vi "read_data.vi"(8 "error in (no error)":errorcluster, 11 "GammaRegressor in":refnum<class "GammaRegressor.lvclass">) -> (0 "error out":errorcluster, 2 "data":T1, 3 "GammaRegressor out":refnum<class "GammaRegressor.lvclass">)   [LabVIEW 2020, in "GammaRegressor.lvclass"]
uses:
  GammaRegressor.lvclass
  Controls/gamma_regressor_data.ctl
  GammaRegressor.lvclass/GammaRegressor.ctl
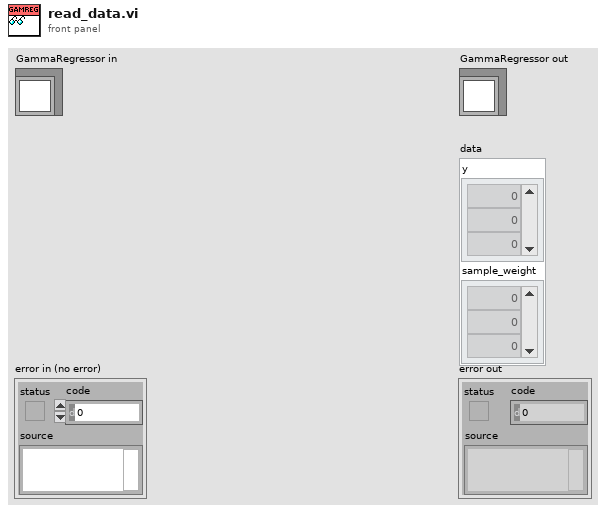
[diagram p1: front panel]
types:
  T1 = typedef "gamma_regressor_data.ctl" = cluster{"y":dbl[], "sample_weight":dbl[]}
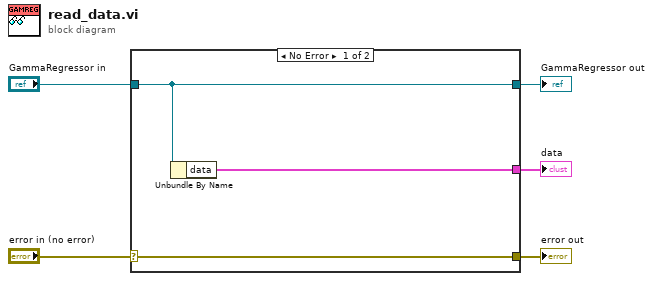
[diagram p0: block diagram]
diagram:
  n1 = case shown="No Error" "error in (no error)" {
    selector: "error in (no error)" -> [w8 w9]
    tunnel: [w8 w9] -> w4
    tunnel: [w7 w10] -> w2
    tunnel: "GammaRegressor in" -> [w7 w10]
    tunnel: [w6 _] -> w1
    frame No Error {
      n2 = Unbundle By Name(w7) -> ("data"=w6:T1)
    }
    frame Error {
    }
  }
  "error out" <- w4
  "GammaRegressor out" <- w2
  "data" <- w1
